vi "CH1_Save_Header_Python.vi"() -> ()   [LabVIEW 2018]
uses:
  RxTx/RxTx.lvclass
  Save Image/Save Image.lvclass
  Channel/Channel.lvclass
panel:
  in  "Stop Button":bool
  out "error out":errorcluster
  in  "Save Image out":refnum<class "Save Image.lvclass">
  in  "RxTx.lvclass":refnum<class "RxTx.lvclass">
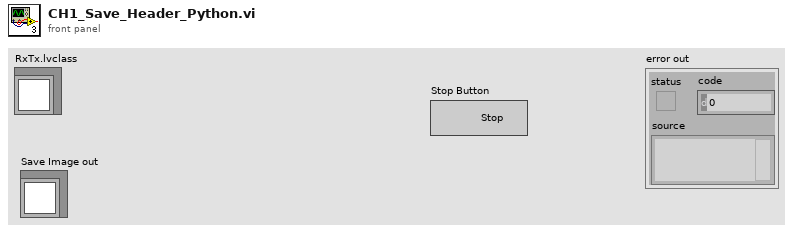
[diagram p1: front panel]
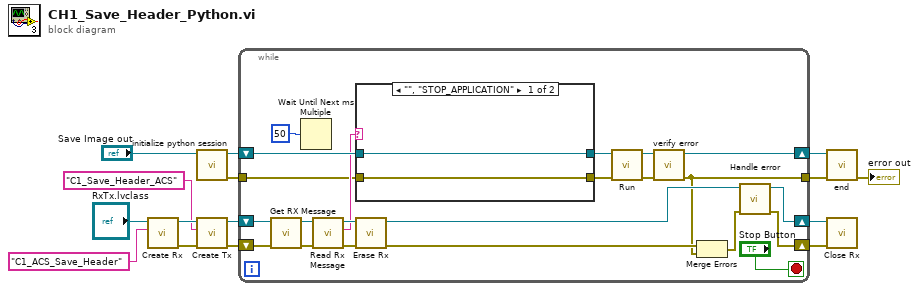
[diagram p0: block diagram]
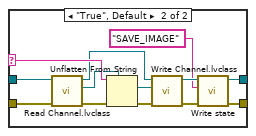
[diagram p2: hidden frame]
diagram:
  n1 = call "Create Rx.vi"("Reader Name"="C1_ACS_Save_Header", "RxTx in"="RxTx.lvclass") -> ("error out"=w8:errorcluster, "RxTx out"=w9:refnum<class "RxTx.lvclass">)  [unwired: 8 in]
  n2 = call "initialize python session.vi"("Save Image in"="Save Image out") -> ("error out"=w5:errorcluster, "Save Image out"=w13:refnum<class "Save Image.lvclass">)  [unwired: 9 in]
  n3 = call "Create Tx.vi"("error in (no error)"=w8, "Writer Name"="C1_Save_Header_ACS" ("Reader Name"), "RxTx in"=w9) -> ("error out"=w1:errorcluster, "RxTx out"=w2:refnum<class "RxTx.lvclass">)  [unwired: 7 in]
  n4 = while {
    shift-right: [w25] -> w6
    shift-left: w2 -> [w37]
    shift-right: [w18] -> w11
    shift-left: w13 -> [w30]
    shift-right: [w24] -> w3
    shift-left: w1 -> [w36]
    tunnel: w5 -> [w26]
    tunnel: [w17] -> w4
    stop <- "Stop Button" stop-if-true
    n5 = call "Get RX Message.vi"("error in (no error)"=w36, "RxTx in"=w37) -> ("error out"=w34:errorcluster, "RxTx out"=w35:refnum<class "RxTx.lvclass">)  [unwired: 7 in, 1 out]
    n6 = Wait Until Next ms Multiple(millisecond multiple=u32 50) -> ()  [unwired: 1 out]
    n7 = call "Read Rx Message.vi"("error in (no error)"=w34, "RxTx in"=w35) -> ("error out"=w28:errorcluster, "Rx Message"=w27:string, "RxTx out"=w29:refnum<class "RxTx.lvclass">)  [unwired: 7 in]
    n8 = case shown="\"\", \"STOP_APPLICATION\"" w27 {
      selector: w27 -> [_ w52]
      tunnel: [w39 w43] -> w32
      tunnel: [w38 w41] -> w31
      tunnel: w26 -> [w38 w50]
      tunnel: w30 -> [w39 w51]
      frame "", "STOP_APPLICATION" {
      }
      frame "True", Default {
        n9 = call-dynamic "Read Channel.lvclass.vi"("error in (no error)"=w50, "Save Image in"=w51) -> ("error out"=w49:errorcluster, "Channel.lvclass"=w46:refnum<class "Channel.lvclass">, "Save Image out"=w47:refnum<class "Save Image.lvclass">)  [unwired: 7 in]
        n10 = Unflatten From String(type=w46, binary string=w52, error in (no error)=w49) -> (value=w45:refnum<class "Channel.lvclass">, error out=w48:errorcluster)  [unwired: 2 in, 1 out]
        n11 = call-dynamic "Write Channel.lvclass.vi"("error in (no error)"=w48, "Channel.lvclass"=w45, "Save Image in"=w47) -> ("error out"=w42:errorcluster, "Save Image out"=w44:refnum<class "Save Image.lvclass">)  [unwired: 7 in]
        n12 = call "Write state.vi"("error in (no error)"=w42, "String"="SAVE_IMAGE" ("Reader Name"), "Save Image in"=w44) -> ("error out"=w41:errorcluster, "Save Image out"=w43:refnum<class "Save Image.lvclass">)  [unwired: 7 in]
      }
    }
    n13 = call "Erase Rx.vi"("error in (no error)"=w28, "RxTx in"=w29) -> ("error out"=w21:errorcluster, "RxTx out"=w23:refnum<class "RxTx.lvclass">)  [unwired: 8 in]
    n14 = call "Run.vi"("error in (no error)"=w31, "Save Image in"=w32) -> ("error out"=w20:errorcluster, "Save Image out"=w19:refnum<class "Save Image.lvclass">)  [unwired: 8 in]
    n15 = call "verify error.vi"("error in (no error)"=w20, "Save Image in"=w19) -> ("error out"=w17:errorcluster, "Save Image out"=w18:refnum<class "Save Image.lvclass">)  [unwired: 8 in]
    n16 = Merge Errors(w21, w17) -> (w22:errorcluster)
    n17 = call "Handle error.vi"("error in (no error)"=w22, "RxTx in"=w23) -> ("error out"=w24:errorcluster, "RxTx out"=w25:refnum<class "RxTx.lvclass">)  [unwired: 8 in]
  }
  n18 = call "end.vi"("error in (no error)"=w4, "Save Image in"=w11) -> ("error out"=→"error out":errorcluster)  [unwired: 8 in, 1 out]
  n19 = call "Close Rx.vi"("error in (no error)"=w3, "RxTx in"=w6) -> ()  [unwired: 8 in, 2 out]
